vi "2D array separate positive negative data.vi"(1 "key row":dbl, 2 "input":dbl[][](array[numeric])) -> (0 "pos and negattive":dbl[][][](array[numeric]))   [LabVIEW 2025]
panel:
  out "key row data":dbl[](graph)
  out "negative 2D array":dbl[][](array[numeric])
  out "positive 2D array":dbl[][](array[numeric])
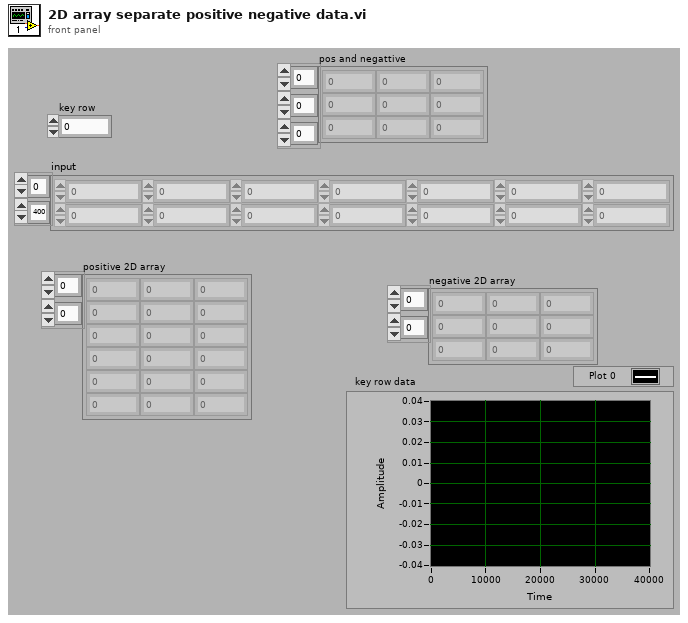
[diagram p1: front panel]
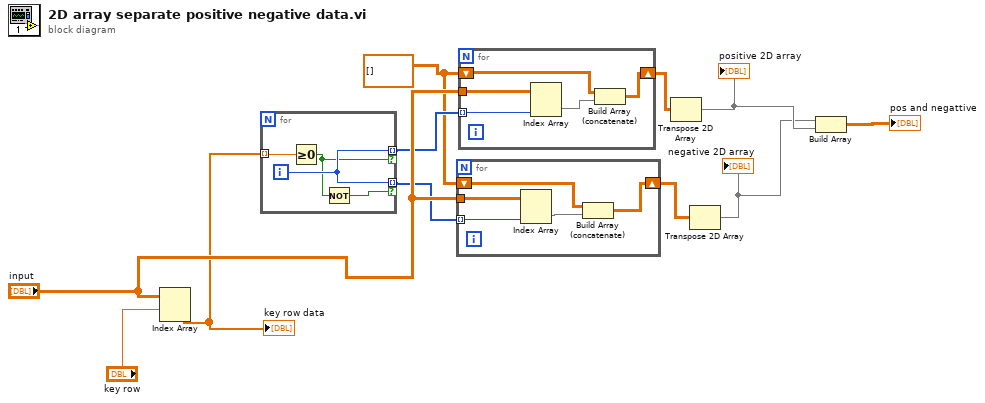
[diagram p0: block diagram]
diagram:
  w7 = dbl[][] []
  n1 = Index Array(array="input", index (row)="key row") -> (element=w3:dbl[])  [unwired: 1 in]
  "key row data" <- w3
  n2 = for {
    tunnel: w3 -> [w15] mode=indexing
    tunnel: [w14] -> w8 mode=indexing if=w12
    tunnel: [w14] -> w9 mode=indexing if=w13
    i -> [w14]
    n3 = Greater Or Equal To 0?(x=w15) -> (x >= 0?=w13:bool)
    n4 = Not(x=w13) -> (.not. x?=w12:bool)
  }
  n5 = for {
    tunnel: "input" -> [w20]
    tunnel: w8 -> [w19] mode=indexing
    shift-right: [w17] -> w6
    shift-left: w7 -> [w16]
    n6 = Index Array(array=w20, index (col)=w19) -> (element=w18:dbl[])  [unwired: 1 in]
    n7 = Build Array (concatenate)(w16, w18) -> (w17:dbl[][])
  }
  n8 = for {
    tunnel: "input" -> [w25]
    tunnel: w9 -> [w24] mode=indexing
    shift-right: [w22] -> w5
    shift-left: w7 -> [w21]
    n9 = Index Array(array=w25, index (col)=w24) -> (element=w23:dbl[])  [unwired: 1 in]
    n10 = Build Array (concatenate)(w21, w23) -> (w22:dbl[][])
  }
  n11 = Transpose 2D Array(2D array=w5) -> (transposed array=w2:dbl[][])
  "positive 2D array" <- w2
  n12 = Transpose 2D Array(2D array=w6) -> (transposed array=w1:dbl[][])
  "negative 2D array" <- w1
  n13 = Build Array(w1, w2) -> (→"pos and negattive":dbl[][][])
